vi "I_Sense_v2.vi"(8 "error in":errorcluster, 9 "Test Freq":enum16{"10Hz", "1kHz", "20kHz"}(ring), 10 "Write Channel(s)":string="NI9264/ao2", 11 "Read Task":string="BONTS_ISENSE") -> (0 "error out":errorcluster, 3 "Result":dbl[](array[numeric]))   [LabVIEW 2021]
uses:
  <vilib>/DAQmx/write.llb/DAQmx Write (Analog 1D Wfm NChan NSamp).vi
  <vilib>/DAQmx/read.llb/DAQmx Read (Analog 1D Wfm NChan NSamp).vi
  <vilib>/DAQmx/create/channels.llb/DAQmx Create Channel (AO-Voltage-Basic).vi
  <vilib>/DAQmx/configure/timing.llb/DAQmx Timing (Sample Clock).vi
  <vilib>/measure/mascope.llb/Amplitude and Levels N chan.vi
  <vilib>/DAQmx/miscellaneous.llb/DAQmx Fill In Error Info.vi
  <vilib>/measure/madcrms.llb/Basic Averaged DC-RMS for N Chan.vi
  <resource>/objmgr/daqmx.rc
  <vilib>/measure/NI_MABase.lvlib
  <vilib>/measure/NI_MAPro.lvlib
panel:
  out "DC values":dbl[](array[numeric]) format="%.2p"
  out "Gains":dbl[](array[numeric])
  out "Amplitude Out":dbl[](array[numeric]) format="%.2p"
  out "High Out":dbl[](array[numeric]) format="%.2p"
  out "Low Out":dbl[](array[numeric]) format="%.2p"
  out "Amplitude In":dbl[](array[numeric]) format="%.2p"
  out "Low In":dbl[](array[numeric]) format="%.2p"
  out "High In":dbl[](array[numeric]) format="%.2p"
  in  "Sample Mode":i32(ring)=10123 items=["Finite Samples"=10178, "Continuous Samples"=10123, "Hardware Timed Single Point"=12522]
  out "Output Waveform":waveform(dbl)[](graph)=[{"t0"=timestamp(0 s since 1904-01-01), "dt"=0.001, "Y"=[]}]
  out "Input Waveform":waveform(dbl)[](graph)=[{"t0"=timestamp(0 s since 1904-01-01), "dt"=0.001, "Y"=[]}]
  in  "Number of Samples":i32=500
  in  "Sample Clock Source":tag="OnboardClock"
  out "Actual Sample Rate":dbl=1000.0 format="%0.2f"
  # "ISENSE_C+"
  # "ISENSE_C-"
  # "ISENSE_C+"
  # "ISENSE_C-"
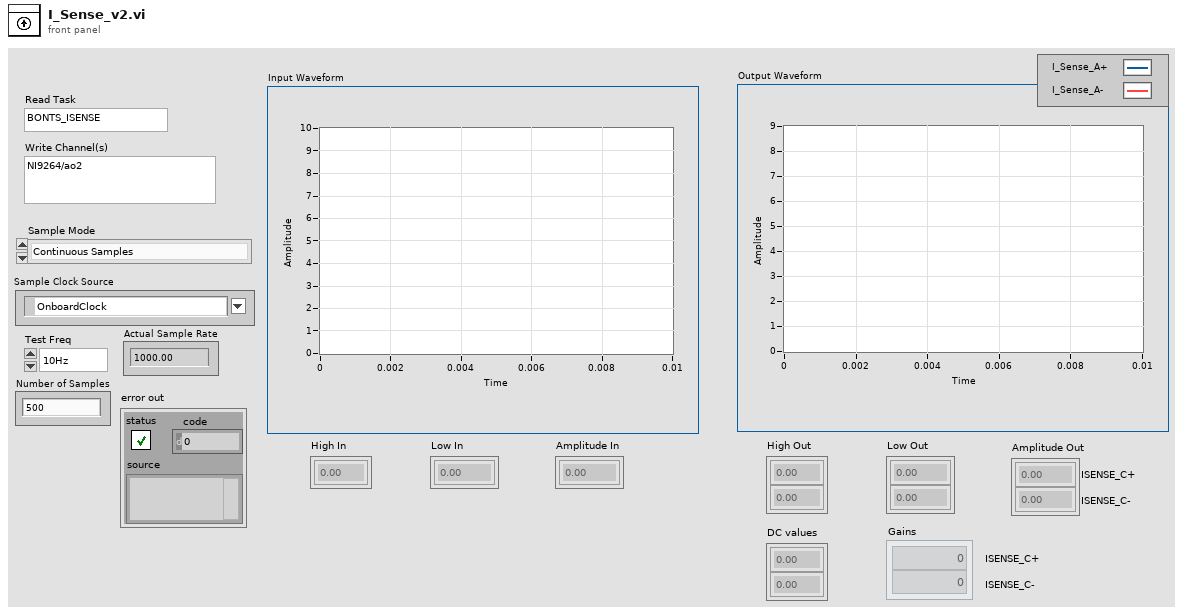
[diagram p1: front panel]
types:
  T1 = cluster{"Waveform Type":u16, "Amplitude":dbl, "Frequency":dbl}[]
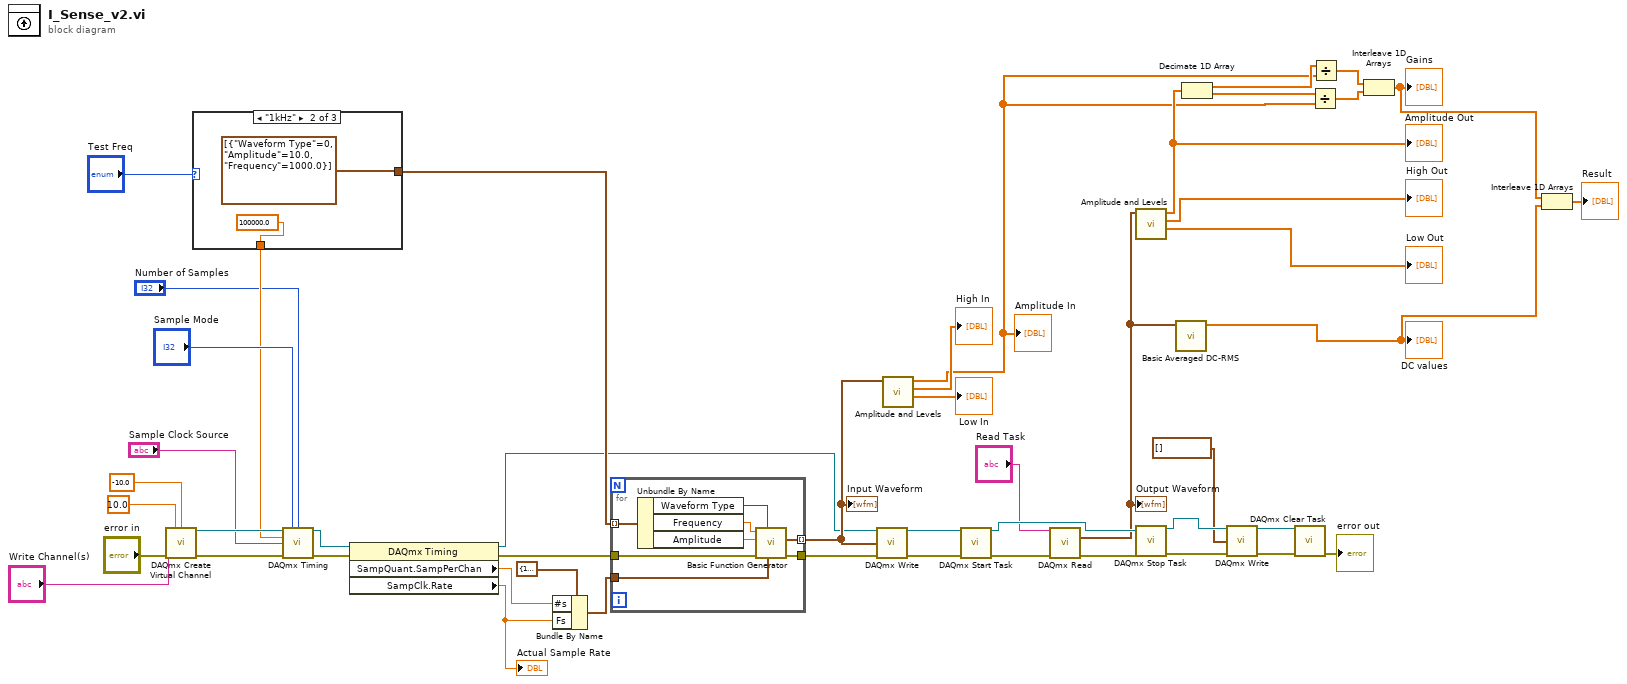
[diagram p0: block diagram]
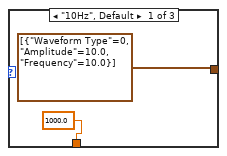
[diagram p2: hidden frame]
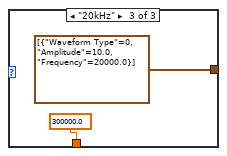
[diagram p3: hidden frame]
diagram:
  n1 = call-poly <vilib>:"DAQmx Create Virtual Channel.vi"("maximum value"=10.0, "minimum value"=-10.0, "physical channels"="Write Channel(s)", "error in"="error in") -> ("task out"=w45:refnum<k21>, "error out"=w46:errorcluster)  [unwired: 10 in]
  n2 = case shown="\"1kHz\"" "Test Freq" {
    tunnel: [1000.0 ("Sample Rate") 100000.0 ("Sample Rate") 300000.0 ("Sample Rate")] -> w43
    tunnel: [T1 [{"Waveform Type"=0, "Amplitude"=10.0, "Frequency"=10.0}] ("Output Array") T1 [{"Waveform Type"=0, "Amplitude"=10.0, "Frequency"=1000.0}] ("Output Array") T1 [{"Waveform Type"=0, "Amplitude"=10.0, "Frequency"=20000.0}] ("Output Array")] -> w37
    frame "10Hz", Default {
    }
    frame "1kHz" {
    }
    frame "20kHz" {
    }
  }
  n3 = call-poly <vilib>:"DAQmx Timing.vi"("task/channels in"=w45, "sample mode"="Sample Mode", "samples per channel"="Number of Samples", "rate"=w43, "source"="Sample Clock Source", "error in"=w46) -> ("task out"=w10:refnum<k21>, "error out"=w48:errorcluster)  [unwired: 8 in]
  n4 = property class="DAQmx Timing"(reference=w10, error in=w48) -> (reference out=w7:refnum<k21>, error out=w32:errorcluster, "SampQuant.SampPerChan"=w35:dbl, "SampClk.Rate"=w34:dbl)
  "Actual Sample Rate" <- w34
  n5 = Bundle By Name(cluster=cluster{"Fs":dbl, "#s":dbl} {"Fs"=1000.0, "#s"=1000.0} ("sampling info"), "#s"=w35, "Fs"=w34) -> (w41:cluster{"Fs":dbl, "#s":dbl})
  n6 = for {
    tunnel: w32 -> [w62]
    tunnel: w41 -> [w61]
    tunnel: [w60] -> w38
    tunnel: w37 -> [w59] mode=indexing
    tunnel: [w55] -> w26 mode=indexing
    n7 = Unbundle By Name(w59) -> ("Waveform Type"=w58:u16, "Frequency"=w57:dbl, "Amplitude"=w56:dbl)
    n8 = call <vilib>:"Basic Function Generator.vi"("sampling info"=w61, "signal type"=w58, "error in (no error)"=w62, "amplitude"=w56, "frequency"=w57) -> ("error out"=w60:errorcluster, "signal out"=w55:waveform(dbl))  [unwired: 4 in, 1 out]
  }
  "Input Waveform" <- w26
  n9 = call-poly <vilib>:"DAQmx Write.vi"("task/channels in"=w7, "data"=w26, "error in"=w38) -> ("task out"=w40:refnum<k21>, "error out"=w39:errorcluster)  [unwired: 10 in, 1 out]
  n10 = call-poly <vilib>:"Amplitude and Levels.vi"("signal(s) in"=w26) -> ("low state level"=→"Low In":dbl[], "high state level"=→"High In":dbl[], "amplitude"=w17:dbl[])  [unwired: 7 in, 1 out]
  "Amplitude In" <- w17
  n11 = call <vilib>:"DAQmx Start Task.vi"("task/channels in"=w40, "error in"=w39) -> ("task out"=w33:refnum<k21>, "error out"=w31:errorcluster)  [unwired: 12 in]
  n12 = call-poly <vilib>:"DAQmx Read.vi"("task/channels in"="Read Task", "error in"=w31) -> ("data"=w14:waveform(dbl)[], "error out"=w30:errorcluster)  [unwired: 11 in, 1 out]
  "Output Waveform" <- w14
  n13 = call-poly <vilib>:"Amplitude and Levels.vi"("signal(s) in"=w14) -> ("low state level"=→"Low Out":dbl[], "high state level"=→"High Out":dbl[], "amplitude"=w20:dbl[])  [unwired: 7 in, 1 out]
  "Amplitude Out" <- w20
  n14 = call <vilib>:"DAQmx Stop Task.vi"("task/channels in"=w33, "error in"=w30) -> ("task out"=w3:refnum<k21>, "error out"=w6:errorcluster)  [unwired: 12 in]
  n15 = call-poly <vilib>:"Basic Averaged DC-RMS.vi"("signals in"=w14) -> ("DC values"=w12:dbl[])  [unwired: 7 in, 3 out]
  "DC values" <- w12
  n16 = Decimate 1D Array(w20) -> (w19:dbl[], w18:dbl[])
  n17 = call-poly <vilib>:"DAQmx Write.vi"("task/channels in"=w3, "data"=waveform(dbl)[] [], "error in"=w6) -> ("task out"=w2:refnum<k21>, "error out"=w5:errorcluster)  [unwired: 10 in, 1 out]
  n18 = call <vilib>:"DAQmx Clear Task.vi"("task in"=w2, "error in"=w5) -> ("error out"=→"error out":errorcluster)  [unwired: 13 in]
  n19 = Divide(x=w18, y=w17) -> (x/y=w15:dbl[])
  n20 = Divide(x=w19, y=w17) -> (x/y=w16:dbl[])
  n21 = Interleave 1D Arrays(w16, w15) -> (w13:dbl[])
  "Gains" <- w13
  n22 = Interleave 1D Arrays(w13, w12) -> (→"Result":dbl[])
